vi "Get-pane-status.vi"(8 "error in (no error)":errorcluster, 10 "Pane":T1, 11 "Panes in":T2) -> (0 "error out":errorcluster, 2 "Status":bool, 3 "Panes out":T2)   [LabVIEW 2013, in "SLMControl.lvlib" / "SC-UI.lvclass"]
uses:
  SC-UI.lvclass
  Panes-reference.ctl
  Pane-names.ctl
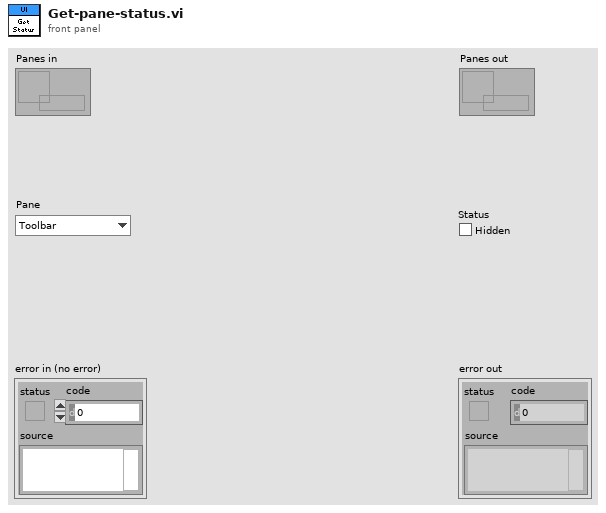
[diagram p1: front panel]
types:
  T1 = typedef "SLMControl.lvlib/SC-UI.lvclass/Pane-names.ctl" = enum16{"Toolbar", "Help bar", "Toolbar lower border", "Center panel", "Main panel", "Status panel", "Status bar upper border", "General state bar", "Information bar"}
  T2 = typedef "SLMControl.lvlib/SC-UI.lvclass/Panes-reference.ctl" = refnum<data-value>
  T3 = typedef "SLMControl.lvlib/SC-UI.lvclass/Pane-settings.ctl" = cluster{"Pane-name":T1, "Startup status":bool, "Current status":bool, "Splitters":T4[], "Pane-reference":refnum<vi>}
  T4 = typedef "SLMControl.lvlib/SC-UI.lvclass/Splitter-settings.ctl" = cluster{"Splitter-name":T5, "Position shown":i32, "Position hidden":i32, "Splitter reference":refnum<vi>}
  T5 = typedef "SLMControl.lvlib/SC-UI.lvclass/Splitter-names.ctl" = enum16{"Upper toolbar splitter", "Help bar splitter", "Lower toolbar splitter", "Upper status bar splitter", "Lower status bar splitter", "Left status bar splitter", "Status splitter"}
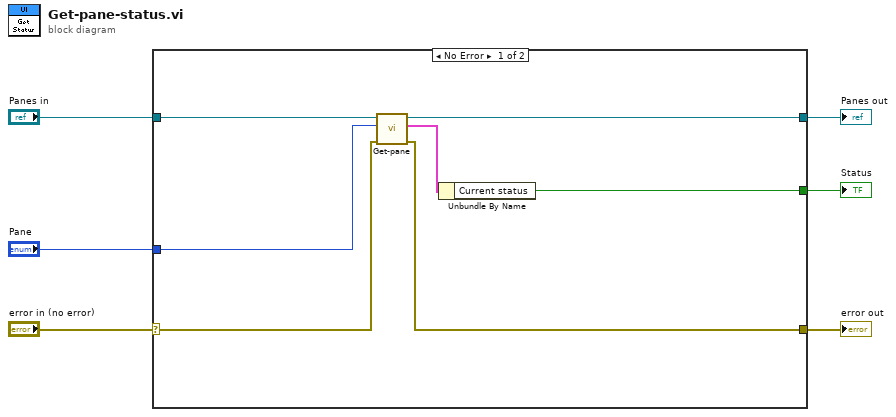
[diagram p0: block diagram]
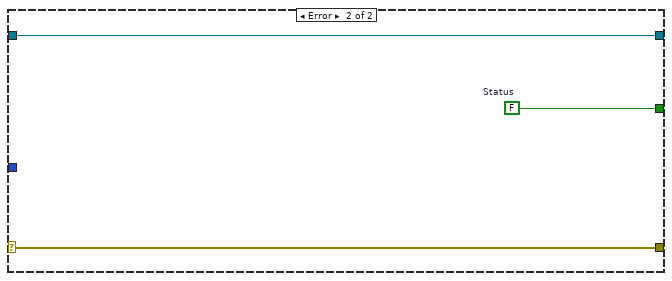
[diagram p2: hidden frame]
diagram:
  n1 = case shown="No Error" "error in (no error)" {
    selector: "error in (no error)" -> [w7 w15]
    tunnel: [w8 w15] -> w5
    tunnel: [w12 w16] -> w3
    tunnel: "Panes in" -> [w13 w16]
    tunnel: "Pane" -> [w11 _]
    tunnel: [w9 w14] -> w1
    frame No Error {
      n2 = call "Get-pane.vi"("error in (no error)"=w7, "Pane"=w11, "Panes in"=w13) -> ("error out"=w8:errorcluster, "Pane"=w10:T3, "Panes out"=w12:T2)  [unwired: 5 in, 1 out]
      n3 = Unbundle By Name(w10) -> ("Current status"=w9:bool)
    }
    frame Error {
      w14 = FALSE  # Status
    }
  }
  "error out" <- w5
  "Panes out" <- w3
  "Status" <- w1
